vi "Read Icon Data from Library.vi"(8 "error in (no error)":errorcluster, 10 "Default body text":T2 {"Body Text Spec"."Alignment" items=["left", "center", "right"]}, 11 "Library in":refnum<vi>) -> (0 "error out":errorcluster, 2 "Data":T1={"Text Visible?"=FALSE, "Text Opacity"=0, "Templ Visible?"=FALSE, "Templ Opacity"=0, "Relative Path from 1 to 2"=path "", "Image"=bytes[0], "All User Layers"=[], "Body Text"={"Line 1 text"="", "Line 2 text"="", "Line 3 text"="", "Line 4 text"="", "Line 1 color"=0, "Line 2 color"=0, "Line 3 color"=0, "Line 4 color"=0, "Body Text Spec"={"Font"="", "Alignment"=0, "Size"=3}, "Center text vertically"=FALSE, "Capitalize Text"=FALSE}} {"Body Text"."Body Text Spec"."Alignment" items=["left", "center", "right"]}, 3 "Library out":refnum<vi>)   [LabVIEW 2021, in "lv_icon.lvlib"]
doc: "Read LabVIEW Icon Data from a Library."
uses:
  <vilib>/LabVIEW Icon API/lv_icon/lv_icon.lvlib
  <vilib>/LabVIEW Icon API/lv_icon/Controls/BodyText.ctl
  <vilib>/LabVIEW Icon API/lv_icon/Controls/Font.ctl
  <vilib>/LabVIEW Icon API/lv_icon/Controls/Alignment.ctl
  <vilib>/LabVIEW Icon API/lv_icon/Controls/LabVIEW Icon Stored Information.ctl
  <vilib>/LabVIEW Icon API/lv_icon/Classes/Layer/Layer.lvclass
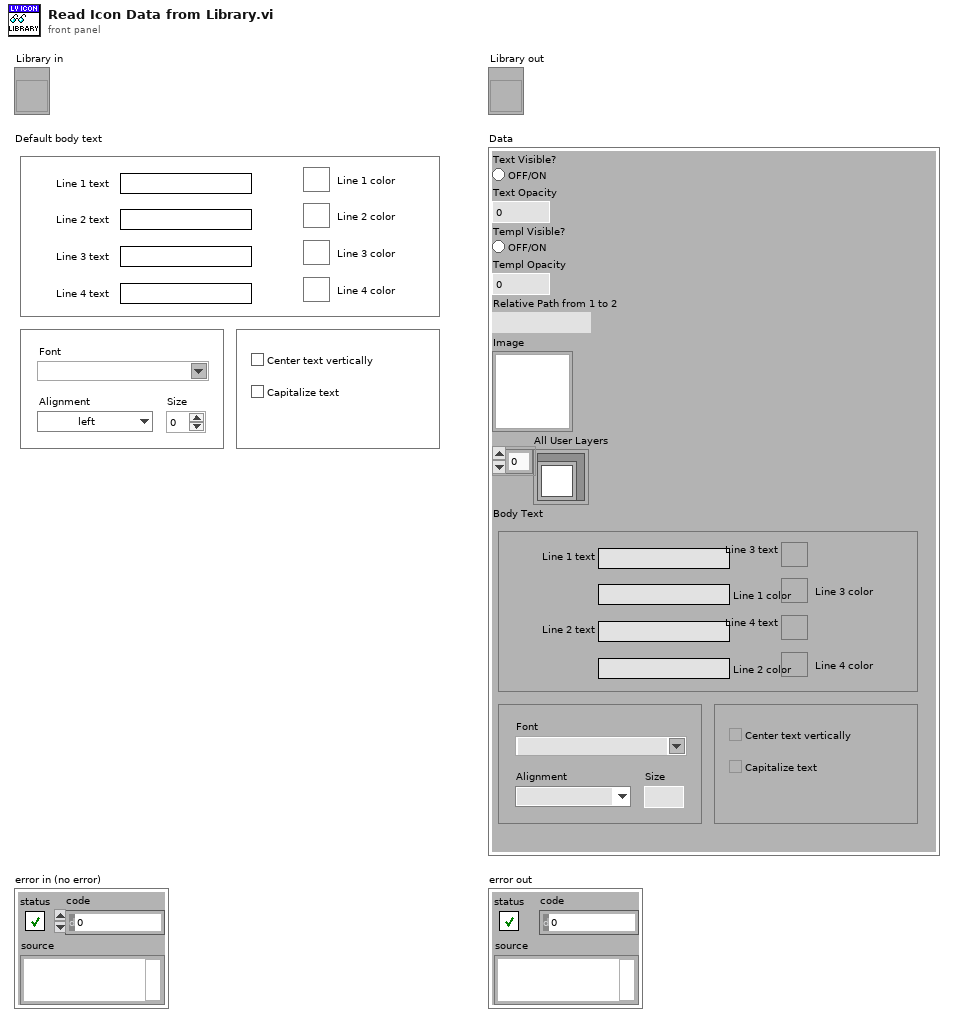
[diagram p1: front panel]
types:
  T1 = typedef "LabVIEW Icon Stored Information.ctl" = cluster{"Text Visible?":bool, "Text Opacity":u8, "Templ Visible?":bool, "Templ Opacity":u8, "Relative Path from 1 to 2":path, "Image":picture, "All User Layers":refnum<class "Layer.lvclass">[], "Body Text":T2}
  T2 = typedef "BodyText.ctl" = cluster{"Line 1 text":string, "Line 2 text":string, "Line 3 text":string, "Line 4 text":string, "Line 1 color":u32, "Line 2 color":u32, "Line 3 color":u32, "Line 4 color":u32, "Body Text Spec":cluster{"Font":T3, "Alignment":T4, "Size":u8}, "Center text vertically":bool, "Capitalize Text":bool}
  T3 = typedef "Font.ctl" = string
  T4 = typedef "Alignment.ctl" = u16
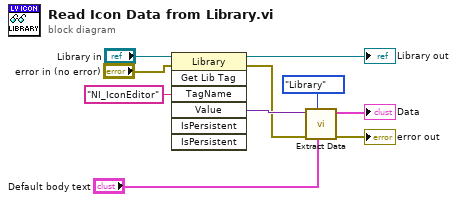
[diagram p0: block diagram]
diagram:
  n1 = invoke class="Library" method="Get Lib Tag"(reference="Library in", error in="error in (no error)", "TagName"="NI_IconEditor" ("Tag Name")) -> (reference out=→"Library out":refnum<vi>, error out=w1:errorcluster, "Value"=w6:variant)  [unwired: 4 in, 4 out]
  n2 = call <vilib>:"Extract Data.vi"("Default body text"="Default body text", "Type"=enum16{"VI", "Library"}."Library", "error in"=w1, "Value"=w6) -> ("error out"=→"error out":errorcluster, "Data"=→"Data":T1)  [unwired: 6 out]
